vi "PPMSDR_MostRecentTwo.vi"(8 "pattern":string="logppmsdata_2016*dat", 9 "directory path":path=path "\\\\PPMS\\Data") -> (2 "String":string)   [LabVIEW 2019]
panel:
  # "List files in a specified folder in order of time stamp.\n\nDaniel L. Press\nPrimeTest Corp.\ndan.press@primetest.com"
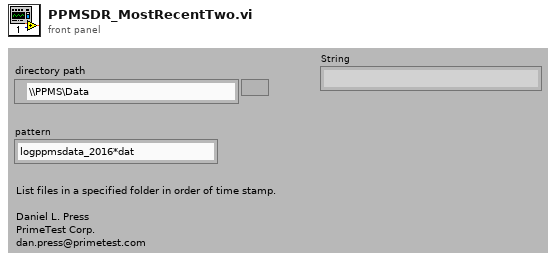
[diagram p1: front panel]
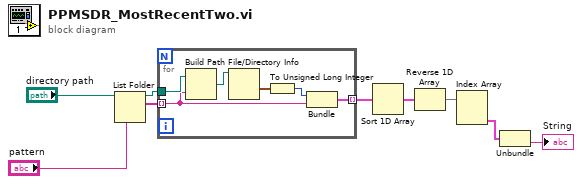
[diagram p0: block diagram]
diagram:
  n1 = List Folder(path="directory path", pattern="pattern") -> (path out=w8:path, filenames=w9:string[])  [unwired: 2 in, 2 out]
  n2 = for {
    tunnel: w9 -> [w11] mode=indexing
    tunnel: w8 -> [w15]
    tunnel: [w13] -> w7 mode=indexing
    n3 = Build Path(base path=w15, name or relative path=w11) -> (appended path=w12:path)
    n4 = File/Directory Info(path=w12) -> (last mod=w10:timestamp)  [unwired: 1 in, 6 out]
    n5 = To Unsigned Long Integer(number=w10) -> (unsigned 32bit integer=w14:u32)
    n6 = Bundle(w14, w11) -> (w13:cluster{u32, string})  [unwired: 1 in]
  }
  n7 = Sort 1D Array(array=w7) -> (sorted array=w5:cluster{u32, string}[])
  n8 = Reverse 1D Array(array=w5) -> (reversed array=w3:cluster{u32, string}[])
  n9 = Index Array(array=w3) -> (element #2=w2:cluster{u32, string})  [unwired: 2 in, 1 out]
  n10 = Unbundle(w2) -> (→"String":string)  [unwired: 1 out]
